vi "Enable RJDJ Clock.vi"(8 "error in (no error)":errorcluster, 10 "Enable RJDJ Clock (F: Disable)":bool, 11 "VISA resource name":refnum<visa-resource-name>) -> (0 "error out":errorcluster, 3 "VISA resource name out":refnum<visa-resource-name>)   [LabVIEW 2020, in "Agilent 90000 Series.lvlib"]
doc: "Enables or disables the RJDJ Clock. \n\n<b>Notes: </b>\n1.This command is available when the EZJIT+ or EZJIT Complete jitter analysis software is installed.\n2. This VI is new in firmware version 4.30."
uses:
  Agilent 90000 Series.lvlib
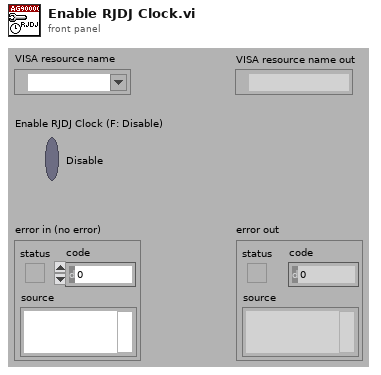
[diagram p1: front panel]
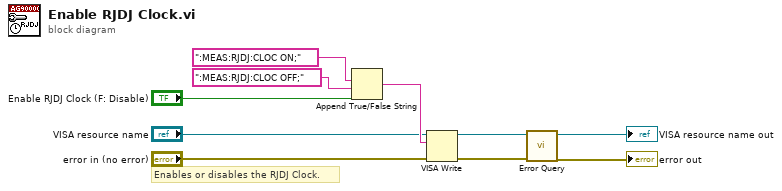
[diagram p0: block diagram]
diagram:
  # "Enables or disables the RJDJ Clock."
  n1 = Append True/False String(1:"Enable RJDJ Clock (F: Disable)", 2:":MEAS:RJDJ:CLOC OFF;", 3:":MEAS:RJDJ:CLOC ON;") -> (0:w7:string)  [unwired: 1 in]
  n2 = VISA Write(VISA resource name="VISA resource name", write buffer=w7, error in (no error)="error in (no error)") -> (VISA resource name out=w4:refnum<visa-resource-name>, error out=w3:errorcluster)  [unwired: 1 out]
  n3 = call "Error Query.vi"("error in (no error)"=w3, "VISA resource name"=w4) -> ("error out"=→"error out":errorcluster, "VISA resource name out"=→"VISA resource name out":refnum<visa-resource-name>)  [unwired: 6 in, 2 out]
